vi "Delete Math Operation.vi"(7 "Delete All Custom Operations (False)":bool, 8 "error in (no error)":errorcluster, 10 "Custom Math Operation Name (\"PCT_DEV\")":string="PCT_DEV", 11 "VISA resource name":refnum<visa-resource-name>) -> (0 "error out":errorcluster, 3 "VISA resource name out":refnum<visa-resource-name>)   [LabVIEW 2021, in "Keithley 24XX.lvlib"]
doc: "Deletes a custom math operation."
uses:
  <instrlib>/Keithley 24XX/Keithley 24XX.lvlib
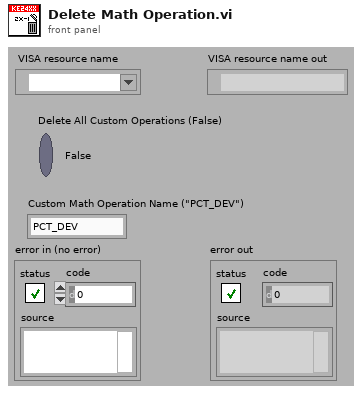
[diagram p1: front panel]
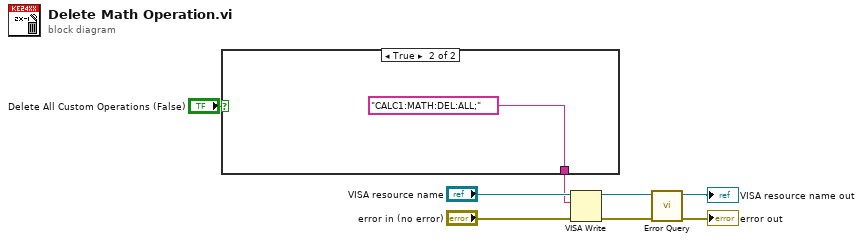
[diagram p0: block diagram]
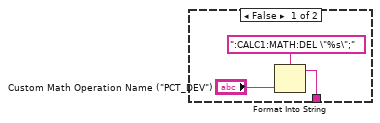
[diagram p2: hidden frame]
diagram:
  n1 = case shown="True" "Delete All Custom Operations (False)" {
    tunnel: [w10 "CALC1:MATH:DEL:ALL;"] -> w2
    frame False {
      n2 = Format Into String(format string=":CALC1:MATH:DEL \"%s\";", "Custom Math Operation Name (\"PCT_DEV\")") -> (resulting string=w10:string)  [unwired: 2 in, 1 out]
    }
    frame True {
    }
  }
  n3 = VISA Write(VISA resource name="VISA resource name", write buffer=w2, error in (no error)="error in (no error)") -> (VISA resource name out=w6:refnum<visa-resource-name>, error out=w3:errorcluster)  [unwired: 1 out]
  n4 = call <instrlib>:"Error Query.vi"("error in (no error)"=w3, "VISA resource name"=w6) -> ("error out"=→"error out":errorcluster, "VISA resource name out"=→"VISA resource name out":refnum<visa-resource-name>)  [unwired: 6 in, 2 out]
